vi "acq_eeg_fin.vi"(8 "error in (no error)":errorcluster, 10 "variant in":variant, 11 "eeg_device":T1) -> (0 "error out":errorcluster)   [LabVIEW 2013]
uses:
  <vilib>/NIOSC/Address Space Node.ctl
  gui/type_def/device.ctl
  <vilib>/NI/Emotiv Toolkit/Emotiv Task.lvclass
  <vilib>/OpenBCI/Comm Protocol/Control Def/openbci_device.ctl
  <vilib>/OpenBCI/Comm Protocol/Control Def/channel_count.ctl
  gui/global_var.vi
  <vilib>/NI/LabVIEW - NeuroSky Driver/NeuroSky Driver.lvlib
  <vilib>/NIOSC/NI_OSC.lvlib
panel:
  in  "NeuroSky Task Out":T2
  in  "muse cluster":T4
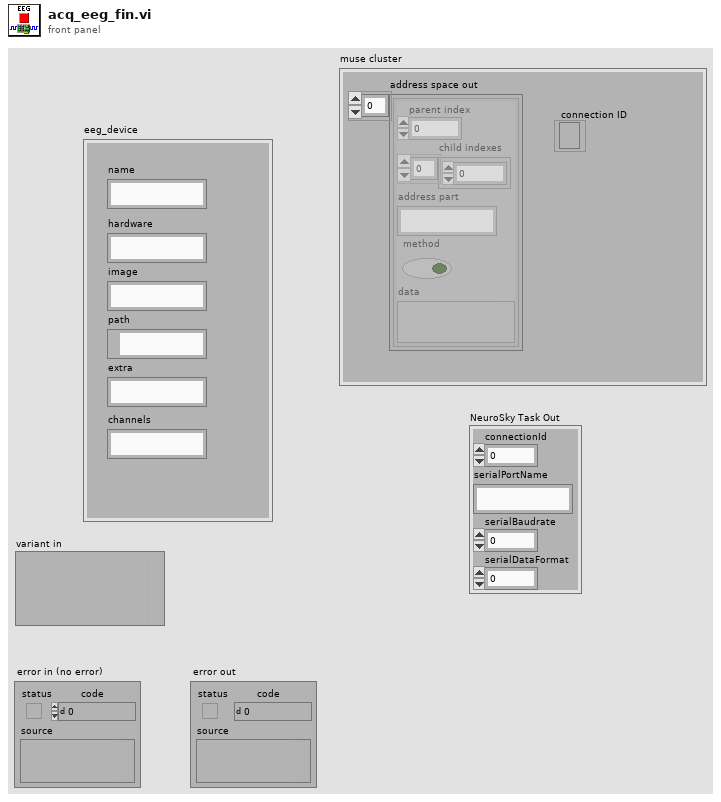
[diagram p1: front panel]
types:
  T1 = typedef "device.ctl" = cluster{"name":string, "hardware":string, "image":string, "path":path, "extra":string, "channels":string}
  T2 = cluster{"connectionId":i32, "serialPortName":string, "serialBaudrate":i32, "serialDataFormat":i32}
  T3 = typedef "NI_OSC.lvlib/Address Space Node.ctl" = cluster{"parent index":i32, "child indexes":i32[], "address part":string, "method":bool, "data":variant}
  T4 = cluster{"address space out":T3[], "connection ID":refnum<k5>}
  T5 = typedef "openbci_device.ctl" = cluster{"COM port":refnum<visa-resource-name>, "n_ch (8)":T6, "delay_tx":u32}
  T6 = typedef "channel_count.ctl" = enum16{"8 Channels", "16 Channels"}
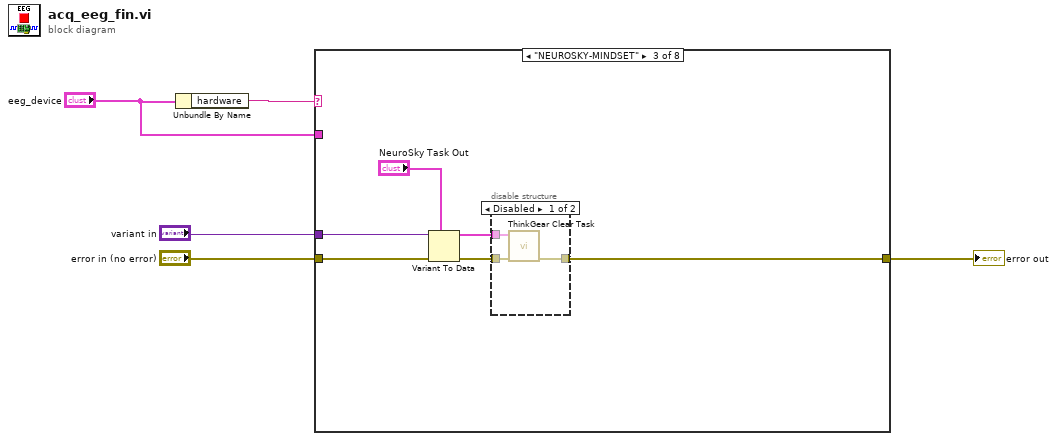
[diagram p0: block diagram]
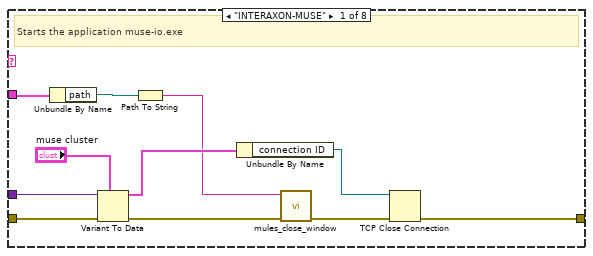
[diagram p2: hidden frame]
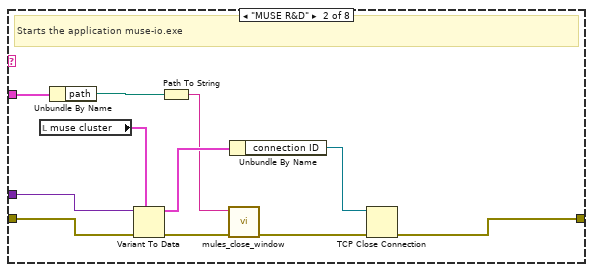
[diagram p3: hidden frame]
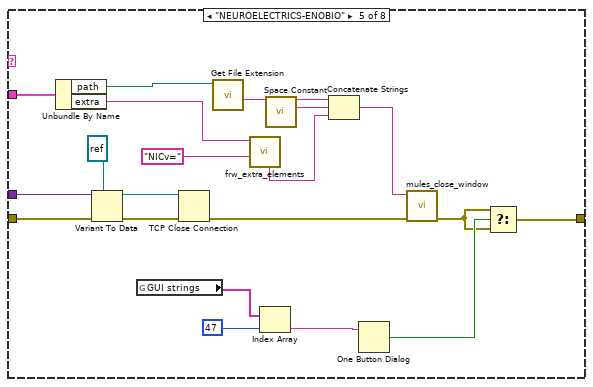
[diagram p6: hidden frame]
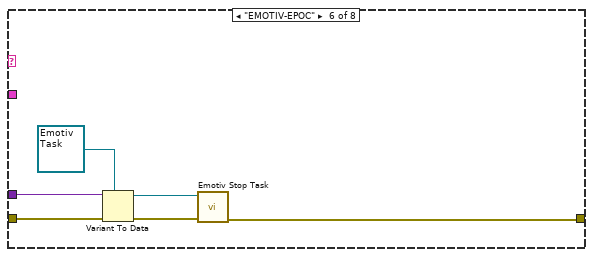
[diagram p7: hidden frame]
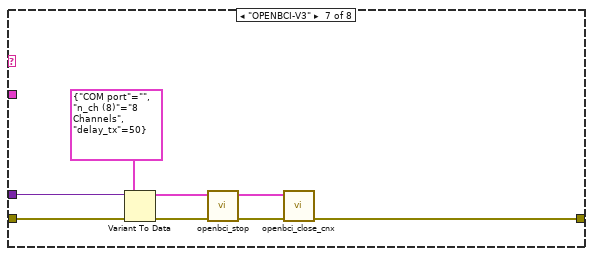
[diagram p8: hidden frame]
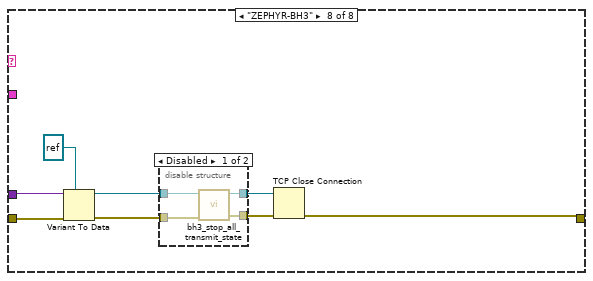
[diagram p9: hidden frame]
diagram:
  n1 = Unbundle By Name("eeg_device") -> ("hardware"=w5:string)
  n2 = case shown="\"NEUROSKY-MINDSET\"" w5 {
    tunnel: "eeg_device" -> [w11 w24 _ _ w52 _ _ _]
    tunnel: "error in (no error)" -> [w9 w22 w32 w37 w54 w61 w68 w78]
    tunnel: [w7 w20 w28 w37 w46 w59 w71 w72] -> w3
    tunnel: "variant in" -> [w15 w26 w31 _ w57 w62 w67 w77]
    frame "INTERAXON-MUSE" {
      # "Starts the application muse-io.exe"
      n3 = Unbundle By Name(w11) -> ("path"=w10:path)
      n4 = Variant To Data(error in=w9, type="muse cluster", Variant=w15) -> (data=w16:T4, error out=w6:errorcluster)
      n5 = Path To String(path=w10) -> (string=w12:string)
      n6 = Unbundle By Name(w16) -> ("connection ID"=w13:refnum<k5>)
      n7 = call "mules_close_window.vi"("error in (no error)"=w6, "IpszWindowName"=w12) -> ("sortie d'erreur"=w8:errorcluster)  [unwired: 9 in]
      n8 = TCP Close Connection(connection ID=w13, error in (no error)=w8) -> (error out=w7:errorcluster)  [unwired: 1 in, 1 out]
    }
    frame "MUSE R&D" {
      # "Starts the application muse-io.exe"
      n9 = local read "muse cluster"() -> (w21:T4)
      n10 = Unbundle By Name(w24) -> ("path"=w23:path)
      n11 = Variant To Data(error in=w22, type=w21, Variant=w26) -> (data=w27:T4, error out=w17:errorcluster)
      n12 = Path To String(path=w23) -> (string=w19:string)
      n13 = call "mules_close_window.vi"("error in (no error)"=w17, "IpszWindowName"=w19) -> ("sortie d'erreur"=w18:errorcluster)  [unwired: 9 in]
      n14 = Unbundle By Name(w27) -> ("connection ID"=w25:refnum<k5>)
      n15 = TCP Close Connection(connection ID=w25, error in (no error)=w18) -> (error out=w20:errorcluster)  [unwired: 1 in, 1 out]
    }
    frame "NEUROSKY-MINDSET" {
      n16 = Variant To Data(error in=w32, type="NeuroSky Task Out", Variant=w31) -> (data=w29:T2, error out=w33:errorcluster)
      n17 = disable-structure shown="Disabled" {
        disable-tunnel: w33 -> [w36 _]
        disable-tunnel: w29 -> [w35 _]
        disable-tunnel: [w34 _] -> w28
        frame Disabled {
          n18 = call <vilib>:"ThinkGear Clear Task.VI"("error in"=w36, "NeuroSky Task In"=w35) -> ("error out"=w34:errorcluster)  [unwired: 9 in]
        }
        frame Enabled {
        }
      }
    }
    frame Default {
    }
    frame "NEUROELECTRICS-ENOBIO" {
      n19 = Unbundle By Name(w52) -> ("path"=w51:path, "extra"=w40:string)
      n20 = Variant To Data(error in=w54, type=refnum<k5> refnum ("connection ID"), Variant=w57) -> (data=w55:refnum<k5>, error out=w53:errorcluster)
      n21 = global read "global_var.vi" "GUI strings"() -> (w42:string[])
      n22 = TCP Close Connection(connection ID=w55, error in (no error)=w53) -> (error out=w47:errorcluster)  [unwired: 1 in, 1 out]
      n23 = call <vilib>:"Get File Extension.vi"("file"=w51) -> ("filename without extension"=w50:string)  [unwired: 7 in, 3 out]
      n24 = call "frw_extra_elements.vi"("single field"="NICv=" ("delimiter (Tab)"), "string"=w40) -> ("single string"=w38:string)  [unwired: 5 in, 4 out]
      n25 = Index Array(array=w42, index=47) -> (element=w41:string)
      n26 = call <vilib>:"Space Constant.vi"() -> ("String"=w49:string)
      n27 = Concatenate Strings(w50, w49, w38) -> (w48:string)
      n28 = One Button Dialog(message=w41) -> (true=w45:bool)  [unwired: 1 in]
      n29 = call "mules_close_window.vi"("error in (no error)"=w47, "IpszWindowName"=w48) -> ("sortie d'erreur"=w44:errorcluster)  [unwired: 9 in]
      n30 = Select(t=w44, s=w45, f=w44) -> (s? t:f=w46:errorcluster)
    }
    frame "EMOTIV-EPOC" {
      n31 = Variant To Data(error in=w61, type=refnum<class "Emotiv Task.lvclass"> refnum ("Emotiv Task in"), Variant=w62) -> (data=w58:refnum<class "Emotiv Task.lvclass">, error out=w60:errorcluster)
      n32 = call <vilib>:"Emotiv Stop Task.vi"("error in (no error)"=w60, "Emotiv Task in"=w58) -> ("error out"=w59:errorcluster)  [unwired: 9 in]
    }
    frame "OPENBCI-V3" {
      n33 = Variant To Data(error in=w68, type=T5 {"COM port"="", "n_ch (8)"=enum."8 Channels", "delay_tx"=50} ("OBCI dev in"), Variant=w67) -> (data=w65:T5, error out=w69:errorcluster)
      n34 = call <vilib>:"openbci_stop.vi"("error in (no error)"=w69, "OBCI dev in"=w65) -> ("error out"=w70:errorcluster, "OBCI dev out"=w64:T5)  [unwired: 8 in]
      n35 = call <vilib>:"openbci_close_cnx.vi"("error in (no error)"=w70, "OBCI dev in"=w64) -> ("error out"=w71:errorcluster)  [unwired: 9 in]
    }
    frame "ZEPHYR-BH3" {
      n36 = Variant To Data(error in=w78, type=refnum<k31> refnum ("bt connection ID in"), Variant=w77) -> (data=w74:refnum<k31>, error out=w75:errorcluster)
      n37 = disable-structure shown="Disabled" {
        disable-tunnel: [w83 _] -> w76
        disable-tunnel: w75 -> [w82 _]
        disable-tunnel: w74 -> [w81 _]
        disable-tunnel: [w80 _] -> w73
        frame Disabled {
          n38 = call <vilib>:"bh3_stop_all_transmit_state.vi"("error in (no error)"=w82, "bt connection ID in"=w81) -> ("error out"=w83:errorcluster, "bt connection ID out"=w80:refnum<k31>)  [unwired: 8 in]
        }
        frame Enabled {
        }
      }
      n39 = TCP Close Connection(connection ID=w73, error in (no error)=w76) -> (error out=w72:errorcluster)  [unwired: 1 in, 1 out]
    }
  }
  "error out" <- w3
